vi "Keithley 6514 Null Reference.vi"(0 "Resource In":refnum<visa-resource-name>, 1 "Check For SCPI Errors? (T)":bool=TRUE, 5 "reference (off:0)":u16(ring) items=["off", "set reference value", "Use Input as Reference"], 7 "reference value (V) (0)":dbl min=-1000000000.0 max=1000000000.0 format="%^.2e", 11 "error in (no error)":T1) -> (4 "Resource Out (dupl)":refnum<visa-resource-name>, 15 "error out":T1)   [LabVIEW 2014, in "KE6514Driver.lvlib"]
doc: "This VI is used to set the Null Reference value.\n\nreference:\n0 = off\n1 = set reference value\n2 = Use Input Signal as reference\n\nreference value:\n-9.999999e20 to +9.999999e20"
uses:
  KE6514Driver.lvlib
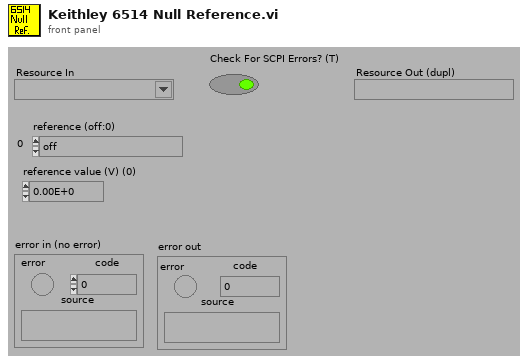
[diagram p1: front panel]
types:
  T1 = cluster{"error":bool, "code":i32, "source":string}
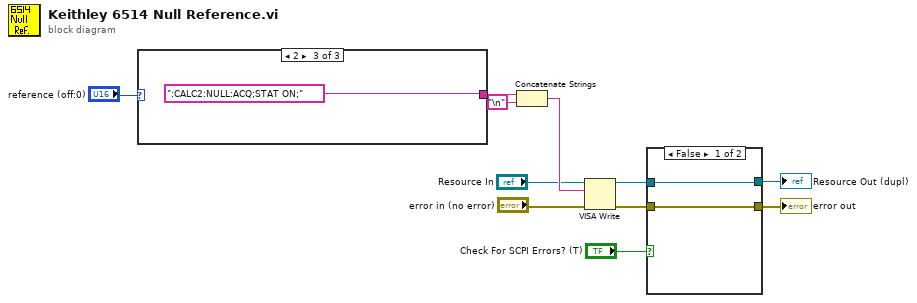
[diagram p0: block diagram]
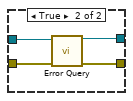
[diagram p2: hidden frame]
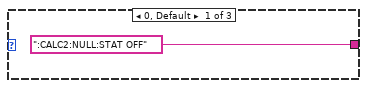
[diagram p3: hidden frame]
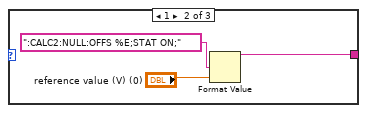
[diagram p4: hidden frame]
diagram:
  n1 = case shown="2" "reference (off:0)" {
    tunnel: [":CALC2:NULL:STAT OFF" w13 ":CALC2:NULL:ACQ;STAT ON;"] -> w10
    frame 0, Default {
    }
    frame 1 {
      n2 = Format Value(format string=":CALC2:NULL:OFFS %E;STAT ON;", value (0)="reference value (V) (0)") -> (output string=w13:string)  [unwired: 1 in]
    }
    frame 2 {
    }
  }
  n3 = Concatenate Strings(w10, "\n") -> (w8:string)
  n4 = VISA Write(VISA resource name="Resource In", write buffer=w8, error in (no error)="error in (no error)") -> (VISA resource name out=w4:refnum<visa-resource-name>, error out=w3:errorcluster)  [unwired: 1 out]
  n5 = case shown="False" "Check For SCPI Errors? (T)" {
    tunnel: w4 -> [w18 w22]
    tunnel: w3 -> [w17 w21]
    tunnel: [w18 w20] -> w2
    tunnel: [w17 w19] -> w1
    frame False {
    }
    frame True {
      n6 = call "Error Query.vi"("VISA Resource In"=w22, "error in (no error)"=w21) -> ("VISA Resource Out (dupl)"=w20:refnum<visa-resource-name>, "error out"=w19:errorcluster)  [unwired: 10 in, 2 out]
    }
  }
  "error out" <- w1
  "Resource Out (dupl)" <- w2
